vi "Read Temperature DBL.vi"(8 "error in":errorcluster, 10 "Source":string, 11 "Virtual Thermometer from CSV in":refnum<class "Virtual Sensor from CSV.lvclass">) -> (0 "error out":errorcluster, 1 "Time Stamp":timestamp format="%<%x %.3X>T", 2 "Temperature":dbl, 3 "Virtual Thermometer from CSV out":refnum<class "Virtual Sensor from CSV.lvclass">)   [LabVIEW 2024, in "Virtual Sensor from CSV.lvclass"]
uses:
  Virtual Sensor from CSV.lvclass
  D:/git/HAL/Source/Action Point/Action Point.lvclass
  Action Point/Action Point.lvclass/Action Point.ctl
  Alarming-Actor/Source/Alarming Actor/Alarming Actor Messages/Update Value Msg/Update Value Msg.lvclass/Update Value Msg.ctl
  <vilib>/ActorFramework/Message Enqueuer/Message Enqueuer.lvclass/Message Enqueuer.ctl
  Action Point/Get Alarming Enqueuer.vi
  Alarming-Actor/Source/Alarming Actor/Alarming Actor Messages/Update Value Msg/Send Update Value.vi
  Action Point/Get Identifier.vi
  <vilib>/ActorFramework/Message Enqueuer/Enqueue.vi
  Alarming-Actor/Source/Alarming Actor/Alarming Actor Messages/Update Value Msg/Update Value Msg.lvclass
  C:/Program Files/National Instruments/LabVIEW 2025/vi.lib/ActorFramework/Message/Message.lvclass
  <vilib>/Utility/LVClass/Get LV Class Name.vi
  <vilib>/ActorFramework/tracing/Trace Generation/Generate Trace for Message.vi
  <vilib>/ActorFramework/Message Priority Queue/Priority Enqueue.vi
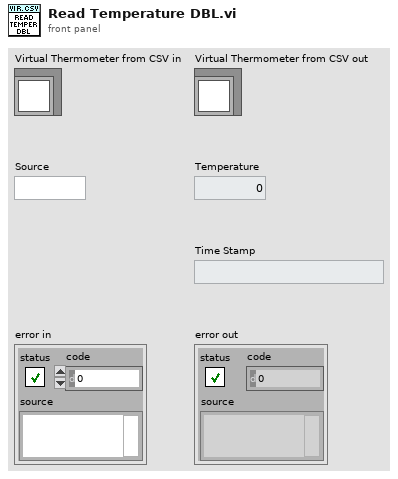
[diagram p1: front panel]
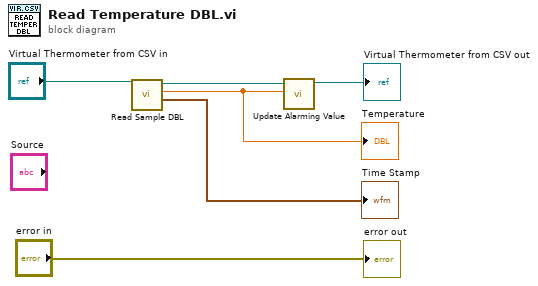
[diagram p0: block diagram]
diagram:
  n1 = call-dynamic "Read Sample DBL.vi"("Virtual Sensor from CSV in"="Virtual Thermometer from CSV in") -> ("Time Stamp"=→"Time Stamp":timestamp, "Sample DBL"=w2:dbl, "Virtual Sensor from CSV out"=w5:refnum<class "Virtual Sensor from CSV.lvclass">)  [unwired: 8 in]
  "Temperature" <- w2
  n2 = call "Update Alarming Value.vi"("Sample DBL"=w2, "Virtual Sensor from CSV in"=w5) -> ("Virtual Sensor from CSV out"=→"Virtual Thermometer from CSV out":refnum<class "Virtual Sensor from CSV.lvclass">)  [unwired: 9 in]
  "error out" <- "error in"
